vi "WLAN_LTF.vi"() -> (3 "LTF":cdb[](array[numeric]))   [LabVIEW 2014]
uses:
  <vilib>/Analysis/2dsp.llb/Inverse Complex FFT.vi
  <vilib>/Analysis/NI_AALPro.lvlib
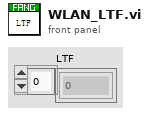
[diagram p1: front panel]
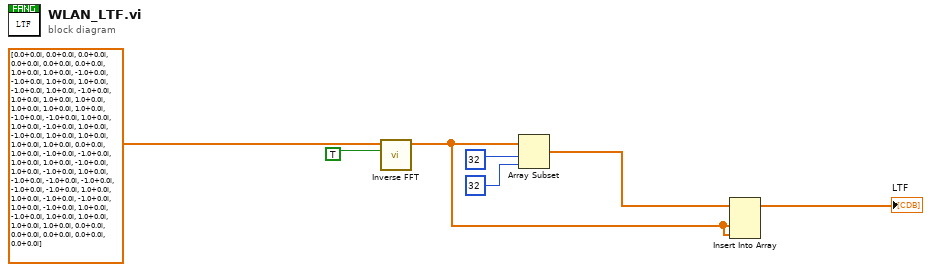
[diagram p0: block diagram]
diagram:
  n1 = call-poly <vilib>:"Inverse FFT.vi"("shift?"=TRUE, "FFT {X}"=cdb[] [0.0+0.0i, 0.0+0.0i, 0.0+0.0i, 0.0+0.0i, 0.0+0.0i, 0.0+0.0i, 1.0+0.0i, 1.0+0.0i, -1.0+0.0i, -1.0+0.0i, 1.0+0.0i, 1.0+0.0i, -1.0+0.0i, 1.0+0.0i, -1.0+0.0i, 1.0+0.0i, 1.0+0.0i, 1.0+0.0i, 1.0+0.0i, 1.0+0.0i, 1.0+0.0i, -1.0+0.0i, -1.0+0.0i, 1.0+0.0i, 1.0+0.0i, -1.0+0.0i, 1.0+0.0i, -1.0+0.0i, 1.0+0.0i, 1.0+0.0i, 1.0+0.0i, 1.0+0.0i, 0.0+0.0i, 1.0+0.0i, -1.0+0.0i, -1.0+0.0i, 1.0+0.0i, 1.0+0.0i, -1.0+0.0i, 1.0+0.0i, -1.0+0.0i, 1.0+0.0i, -1.0+0.0i, -1.0+0.0i, -1.0+0.0i, -1.0+0.0i, -1.0+0.0i, 1.0+0.0i, 1.0+0.0i, -1.0+0.0i, -1.0+0.0i, 1.0+0.0i, -1.0+0.0i, 1.0+0.0i, -1.0+0.0i, 1.0+0.0i, 1.0+0.0i, 1.0+0.0i, 1.0+0.0i, 0.0+0.0i, 0.0+0.0i, 0.0+0.0i, 0.0+0.0i, 0.0+0.0i]) -> ("X"=w2:cdb[])  [unwired: 8 in, 1 out]
  n2 = Array Subset(array=w2, index=32, length=32) -> (w3:cdb[])
  n3 = Insert Into Array(array=w3, new element #1=w2, new element #2=w2) -> (→"LTF":cdb[])  [unwired: 1 in]
